vi "graphe 3.vi"() -> ()   [LabVIEW 2019]
panel:
  out "Waveform Graph":dbl[](graph)
  out "XY Graph":cluster{dbl[], dbl[]}(graph)
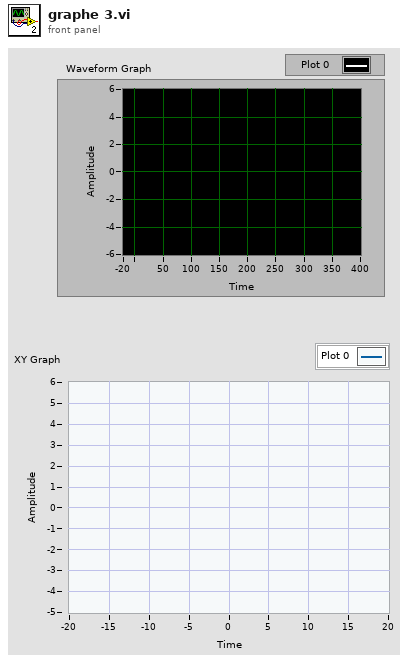
[diagram p1: front panel]
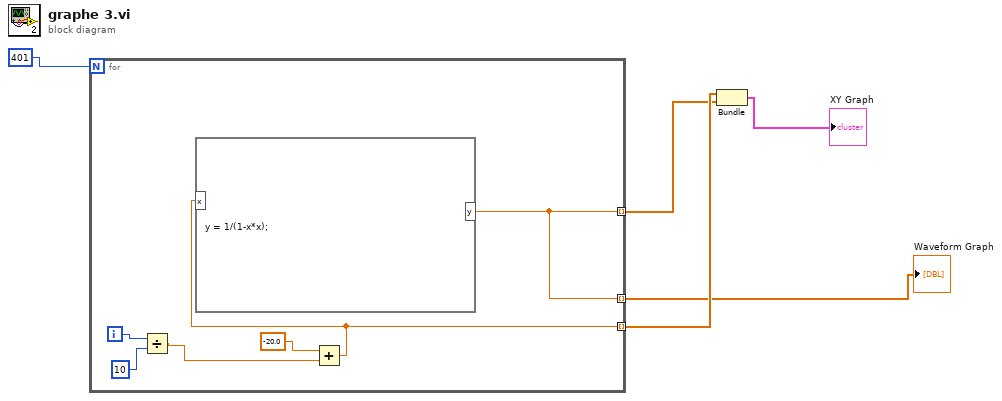
[diagram p0: block diagram]
diagram:
  n1 = for {
    N: 401 -> [_]
    tunnel: [w10] -> w4 mode=indexing
    tunnel: [w9] -> w3 mode=indexing
    tunnel: [w9] -> w1 mode=indexing
    i -> [w8]
    n2 = Divide(x=w8, y=10) -> (x/y=w6:dbl)
    n3 = Add(x=-20.0, y=w6) -> (x+y=w10:dbl)
    n4 = formula code="y = 1/(1-x*x);"("x"=w10) -> ("y"=w9:dbl)
  }
  "Waveform Graph" <- w1
  n5 = Bundle(w4, w3) -> (→"XY Graph":cluster{dbl[], dbl[]})  [unwired: 1 in]
